vi "PH_gentec_P-Link.range 2 limit.vi"(1 "Range":T1 items=["1f", "3f", "10f", "30f", "100f", "300f", "1p", "3p", "10p", "30p", "100p", "300p", "1n", "3n", "10n", "30n", "100n", "300n", "1u", "3u", "10u", "30u", "100u", "300u", "1m", "3m", "10m", "30m", "100m", "300m", "1", "3", "10", "30", "100", "300", "1K", "3K", "10K", "30K", "100K", "300K", "1M", "3M", "10M", "30M", "100M", "300M"]) -> (0 "limit":dbl)   [LabVIEW 2014, in "PH_gentec_P-Link.lvlib"]
doc: "This VI calculates from the range chosen the upper energy value."
uses:
  instr.lib/Gentec-M-Link/Driver/Type Defs/gentec-M-Link.Range.ctl
  PH_gentec_P-Link.lvlib
  instr.lib/Gentec-M-Link/gentec-M-Link - Driver.lvlib
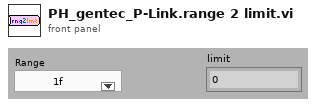
[diagram p1: front panel]
types:
  T1 = typedef "gentec-M-Link - Driver.lvlib/gentec-M-Link.Range.ctl" = u16
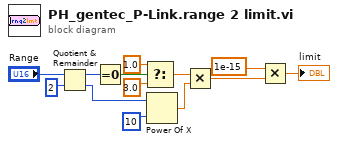
[diagram p0: block diagram]
diagram:
  n1 = Quotient & Remainder(x="Range", y=2) -> (x-y*floor(x/y)=w6:i32, floor(x/y)=w5:i32)
  n2 = Equal To 0?(x=w6) -> (x = 0?=w4:bool)
  n3 = Select(t=1.0, s=w4, f=3.0 ("x/y")) -> (s? t:f=w3:dbl)
  n4 = Power Of X(1:10 ("x"), 2:w5) -> (0:w10:dbl)
  n5 = Multiply(x=w3, y=w10) -> (x*y=w8:dbl)
  n6 = Multiply(x=1e-15, y=w8) -> (x*y=→"limit":dbl)
